vi "SamplesData.vi"() -> ()   [LabVIEW 2012]
panel:
  in  "MeasuresData":T1(array[cluster])
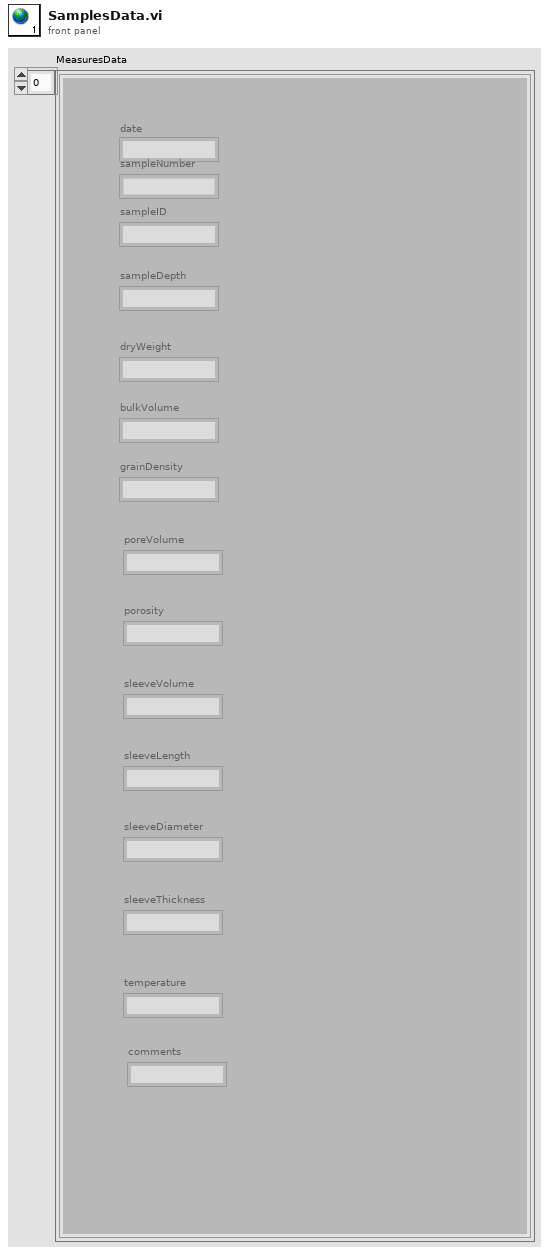
[diagram p1: front panel]
types:
  T1 = cluster{"date":string, "sampleNumber":string, "sampleID":string, "sampleDepth":string, "dryWeight":string, "grainDensity":string, "bulkVolume":string, "poreVolume":string, "porosity":string, "sleeveVolume":string, "sleeveLength":string, "sleeveDiameter":string, "sleeveThickness":string, "temperature":string, "comments":string}[]
diagram:
